vi "process_analysis.vi"(8 "error in (no error)":errorcluster) -> (0 "error out":errorcluster)   [LabVIEW 2010]
uses:
  typedefs/analysis_cluster_dual_channel.ctl
  typedefs/analysis_cluster.ctl
  typedefs/control_analysis_enum.ctl
  typedefs/data_array.ctl
  typedefs/analysis_channels_array.ctl
  typedefs/experiment_mode_enum.ctl
panel:
  in  "What to store":enum32{"Raw data", "Analyzed data"}(radio)
  out "Analysis":T1
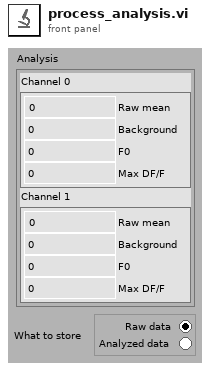
[diagram p1: front panel]
types:
  T1 = typedef "analysis_cluster_dual_channel.ctl" = cluster{"Channel 0":T2, "Channel 1":T2}
  T2 = typedef "analysis_cluster.ctl" = cluster{"Raw mean":dbl, "Background":dbl, "F0":dbl, "Max DF/F":dbl}
  T3 = typedef "analysis_channels_array.ctl" = T2[]
  T4 = typedef "data_array.ctl" = waveform(dbl)[]
  T5 = typedef "control_analysis_enum.ctl" = enum16{"Init", "Analyze", "Reset", "Stop", "Quit"}
  T6 = cluster{"Control Analysis Enum":T5, "variant":variant}
  T7 = cluster{"Data_to_Display_Queue":refnum<queue>, "Data_to_Storage_Queue":refnum<queue>}
  T8 = typedef "experiment_mode_enum.ctl" = enum32{"Raw data", "Measure background", "Measure F0", "Measure DF/F"}
  T9 = cluster{"Experiment mode":T8, "Pixels to integrate":i32, "#channels":i32, "Iteration":i32}
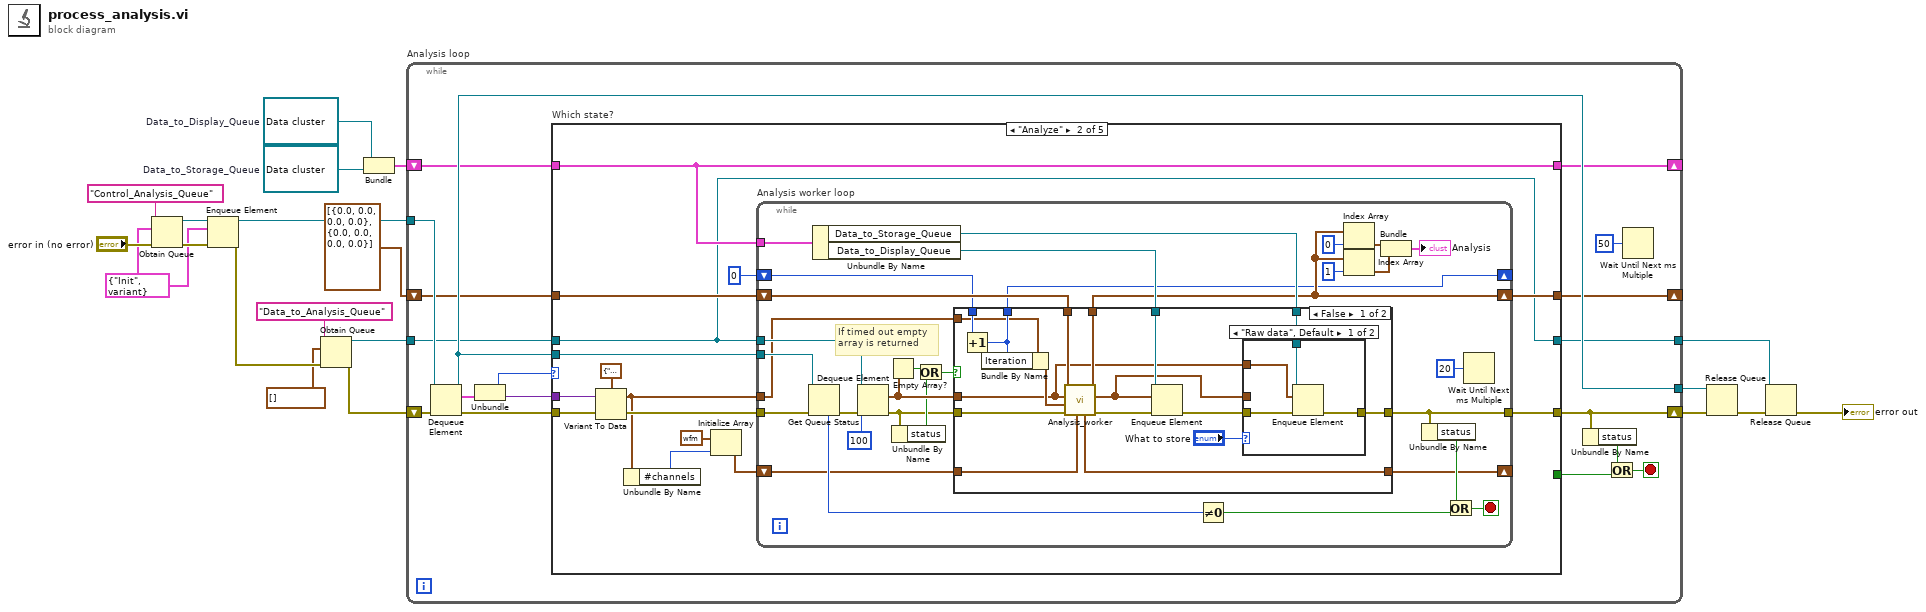
[diagram p0: block diagram]
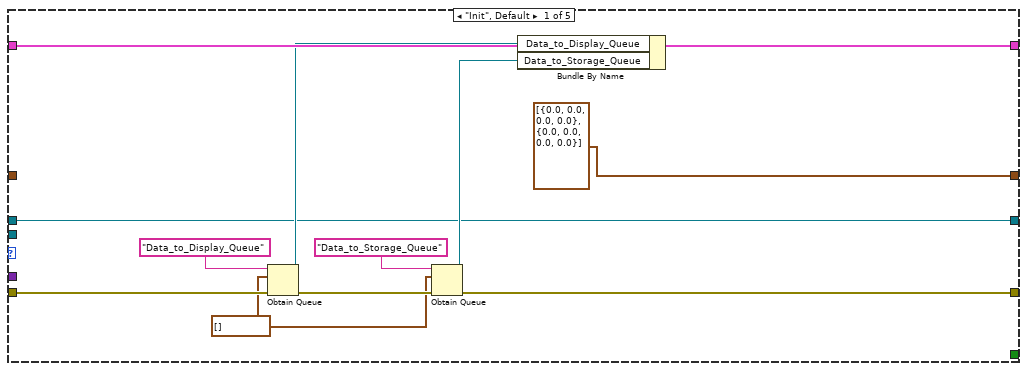
[diagram p2: hidden frame]
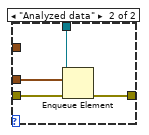
[diagram p3: hidden frame]
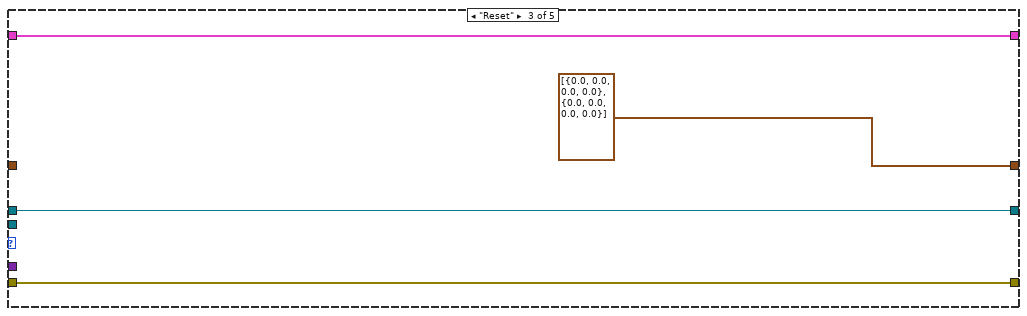
[diagram p5: hidden frame]
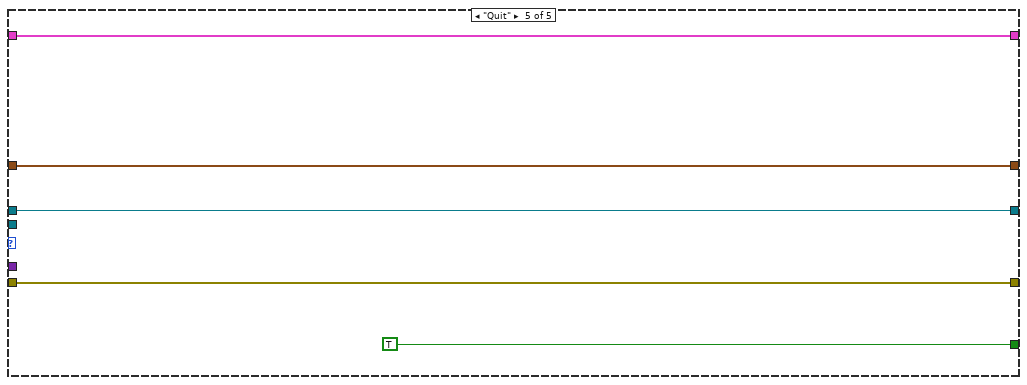
[diagram p7: hidden frame]
diagram:
  w2 = refnum<queue> refnum  # Data_to_Storage_Queue
  w3 = refnum<queue> refnum  # Data_to_Display_Queue
  w16 = T6 {"Control Analysis Enum"=enum."Init", "variant"=variant}
  n1 = Obtain Queue(name (unnamed)="Control_Analysis_Queue", element data type=w16, error in (no error)="error in (no error)") -> (queue out=w17:refnum<queue>, error out=w18:errorcluster)  [unwired: 2 in, 1 out]
  n2 = Enqueue Element(queue=w17, element=w16, error in (no error)=w18) -> (queue out=w15:refnum<queue>, error out=w11:errorcluster)  [unwired: 1 in, 1 out]
  n3 = Obtain Queue(name (unnamed)="Data_to_Analysis_Queue", element data type=T4 [] ("Data cluster"), error in (no error)=w11) -> (queue out=w9:refnum<queue>, error out=w10:errorcluster)  [unwired: 2 in, 1 out]
  n4 = Bundle("Data_to_Display_Queue"=w3, "Data_to_Storage_Queue"=w2) -> (w8:T7)  [unwired: 1 in]
  n5 = while "Analysis loop" {
    shift-right: [w33] -> w14
    shift-left: w10 -> [w35]
    tunnel: w15 -> [w36]
    tunnel: [w28] -> w13
    tunnel: w9 -> [w21]
    shift-right: [w26] -> _
    shift-left: w8 -> [w27]
    tunnel: [w25] -> w5
    shift-right: [w23] -> _
    shift-left: T3 [{"Raw mean"=0.0, "Background"=0.0, "F0"=0.0, "Max DF/F"=0.0}, {"Raw mean"=0.0, "Background"=0.0, "F0"=0.0, "Max DF/F"=0.0}] ("Analysis out") -> [w24]
    stop <- w37 stop-if-true
    n6 = Dequeue Element(queue=w36, error in (no error)=w35) -> (queue out=w28:refnum<queue>, element=w32:T6, error out=w34:errorcluster)  [unwired: 1 in, 1 out]
    n7 = Unbundle(w32) -> ("Control Analysis Enum"=w31:T5, "variant"=w30:variant)
    n8 = case "Which state?" shown="\"Analyze\"" w31 {
      tunnel: w34 -> [w50 w62 w127 w133 w138]
      tunnel: [w45 w65 w127 w133 w138] -> w33
      tunnel: w30 -> [_ w60 _ _ _]
      tunnel: [_ _ _ _ TRUE] -> w29
      tunnel: w28 -> [_ w64 _ _ _]
      tunnel: w27 -> [w48 w63 w129 w132 w136]
      tunnel: [w47 w63 w129 w132 w136] -> w26
      tunnel: [w41 w51 w128 w131 w135] -> w25
      tunnel: w24 -> [_ w58 _ w130 w134]
      tunnel: [T3 [{"Raw mean"=0.0, "Background"=0.0, "F0"=0.0, "Max DF/F"=0.0}, {"Raw mean"=0.0, "Background"=0.0, "F0"=0.0, "Max DF/F"=0.0}] ("Analysis out") w59 T3 [{"Raw mean"=0.0, "Background"=0.0, "F0"=0.0, "Max DF/F"=0.0}, {"Raw mean"=0.0, "Background"=0.0, "F0"=0.0, "Max DF/F"=0.0}] ("Analysis out") w130 w134] -> w23
      tunnel: w21 -> [w41 w51 w128 w131 w135]
      frame "Init", Default {
        w40 = T4 [] ("Data cluster")
        n9 = Obtain Queue(name (unnamed)="Data_to_Display_Queue", element data type=w40, error in (no error)=w50) -> (queue out=w43:refnum<queue>, error out=w46:errorcluster)  [unwired: 2 in, 1 out]
        n10 = Obtain Queue(name (unnamed)="Data_to_Storage_Queue", element data type=w40, error in (no error)=w46) -> (queue out=w42:refnum<queue>, error out=w45:errorcluster)  [unwired: 2 in, 1 out]
        n11 = Bundle By Name(cluster=w48, "Data_to_Display_Queue"=w43, "Data_to_Storage_Queue"=w42) -> (w47:T7)
      }
      frame "Analyze" {
        n12 = Variant To Data(error in=w62, Variant=w60, type=T9 {"Experiment mode"=enum."Raw data", "Pixels to integrate"=0, "#channels"=0, "Iteration"=0} ("output cluster")) -> (error out=w61:errorcluster, data=w55:T9)
        n13 = Unbundle By Name(w55) -> ("#channels"=w54:i32)
        n14 = Initialize Array(waveform(dbl) {"t0"=timestamp(3376681200 s since 1904-01-01), "dt"=1.0, "Y"=[]} ("Waveform"), w54) -> (w52:waveform(dbl)[])
        n15 = while "Analysis worker loop" {
          tunnel: w61 -> [w95]
          tunnel: [w87] -> w65
          tunnel: w64 -> [w93]
          tunnel: w63 -> [w88]
          tunnel: w51 -> [w96]
          tunnel: w55 -> [w68]
          shift-right: [w80] -> w59
          shift-left: w58 -> [w84]
          shift-right: [w81] -> _
          shift-left: w52 -> [w82]
          shift-right: [w66] -> _
          shift-left: 0 -> [w67]
          stop <- w89 stop-if-true
          # "If timed out empty\narray is returned"
          n16 = Get Queue Status(queue=w93, error in (no error)=w95) -> (error out=w94:errorcluster, # elements in queue=w92:i32)  [unwired: 1 in, 6 out]
          n17 = Unbundle By Name(w88) -> ("Data_to_Storage_Queue"=w85:refnum<queue>, "Data_to_Display_Queue"=w86:refnum<queue>)
          n18 = Dequeue Element(queue=w96, timeout in ms (-1)=100, error in (no error)=w94) -> (element=w73:T4, error out=w69:errorcluster)  [unwired: 2 out]
          n19 = Empty Array?(array=w73) -> (empty?=w72:bool)
          n20 = Unbundle By Name(w69) -> ("status"=w71:bool)
          n21 = Or(x=w72, y=w71) -> (x .or. y?=w70:bool)
          n22 = case shown="False" w70 {
            tunnel: [w113 w123] -> w87
            tunnel: w86 -> [w112 _]
            tunnel: w85 -> [w111 _]
            tunnel: [w110 w125] -> w80
            tunnel: w84 -> [w109 w125]
            tunnel: w73 -> [w98 _]
            tunnel: w82 -> [w105 w124]
            tunnel: [w104 w124] -> w81
            tunnel: w68 -> [w100 _]
            tunnel: w69 -> [w103 w123]
            tunnel: w67 -> [w102 w122]
            tunnel: [w101 w122] -> w66
            frame False {
              n23 = Increment(x=w102) -> (x+1=w101:i32)
              n24 = Bundle By Name(cluster=w100, "Iteration"=w101) -> (w99:T9)
              n25 = call "Analysis_worker.vi"("Leftover data in"=w105, "error in"=w103, "Analysis parameters"=w99, "Data in"=w98, "Analysis in"=w109) -> ("error out"=w107:errorcluster, "Data out"=w97:T4, "Analysis out"=w110:T3, "Leftover data out"=w104:T4)  [unwired: 1 in]
              n26 = Enqueue Element(queue=w112, element=w97, error in (no error)=w107) -> (error out=w108:errorcluster)  [unwired: 1 in, 2 out]
              n27 = case shown="\"Raw data\", Default" "What to store" {
                tunnel: [w116 w121] -> w113
                tunnel: w111 -> [w115 w120]
                tunnel: w108 -> [w117 w119]
                tunnel: w97 -> [_ w118]
                tunnel: w98 -> [w114 _]
                frame "Raw data", Default {
                  n28 = Enqueue Element(queue=w115, element=w114, error in (no error)=w117) -> (error out=w116:errorcluster)  [unwired: 1 in, 2 out]
                }
                frame "Analyzed data" {
                  n29 = Enqueue Element(queue=w120, element=w118, error in (no error)=w119) -> (error out=w121:errorcluster)  [unwired: 1 in, 2 out]
                }
              }
            }
            frame True {
            }
          }
          n30 = Not Equal To 0?(x=w92) -> (x != 0?=w91:bool)
          n31 = Index Array(array=w80, index=0) -> (element=w76:T2)
          n32 = Index Array(array=w80, index=1) -> (element=w75:T2)
          n33 = Bundle("Analysis"=w76, "Analysis"=w75) -> (→"Analysis":cluster{"Analysis":T2, "Analysis":T2})  [unwired: 1 in]
          n34 = Unbundle By Name(w87) -> ("status"=w90:bool)
          n35 = Or(x=w90, y=w91) -> (x .or. y?=w89:bool)
          n36 = Wait Until Next ms Multiple(millisecond multiple=u32 20) -> ()  [unwired: 1 out]
        }
      }
      frame "Reset" {
      }
      frame "Stop" {
      }
      frame "Quit" {
      }
    }
    n37 = Unbundle By Name(w33) -> ("status"=w38:bool)
    n38 = Or(x=w38, y=w29) -> (x .or. y?=w37:bool)
    n39 = Wait Until Next ms Multiple(millisecond multiple=u32 50) -> ()  [unwired: 1 out]
  }
  n40 = Release Queue(queue=w13, error in (no error)=w14) -> (error out=w7:errorcluster)  [unwired: 1 in, 2 out]
  n41 = Release Queue(queue=w5, error in (no error)=w7) -> (error out=→"error out":errorcluster)  [unwired: 1 in, 2 out]
